vi "Normalizer.vi"(0 "Acc":u64[][](array[numeric]), 1 "m":dbl, 4 "p":dbl, 5 "Tamaño Sn":i32[](array[numeric]), 6 "Analysis 2":u16(ring) items=["Auto correlation A", "Auto correlation B", "Cross correlation AxB", "Cross correlation BxA"], 7 "AvgA":dbl, 10 "DataA":sgl[](array[numeric]), 11 "AvgB":dbl, 12 "DataB":sgl[](array[numeric])) -> (14 "g(k)":dbl[][](array[numeric]), 18 "s(k)":dbl[][](array[numeric]))   [LabVIEW 2015]
panel:
  out "X2Tau":dbl[][](array[numeric])
  out "X2i":dbl[][](array[numeric])
  out "element":i32
  out "size(s)":i32[](array[numeric])
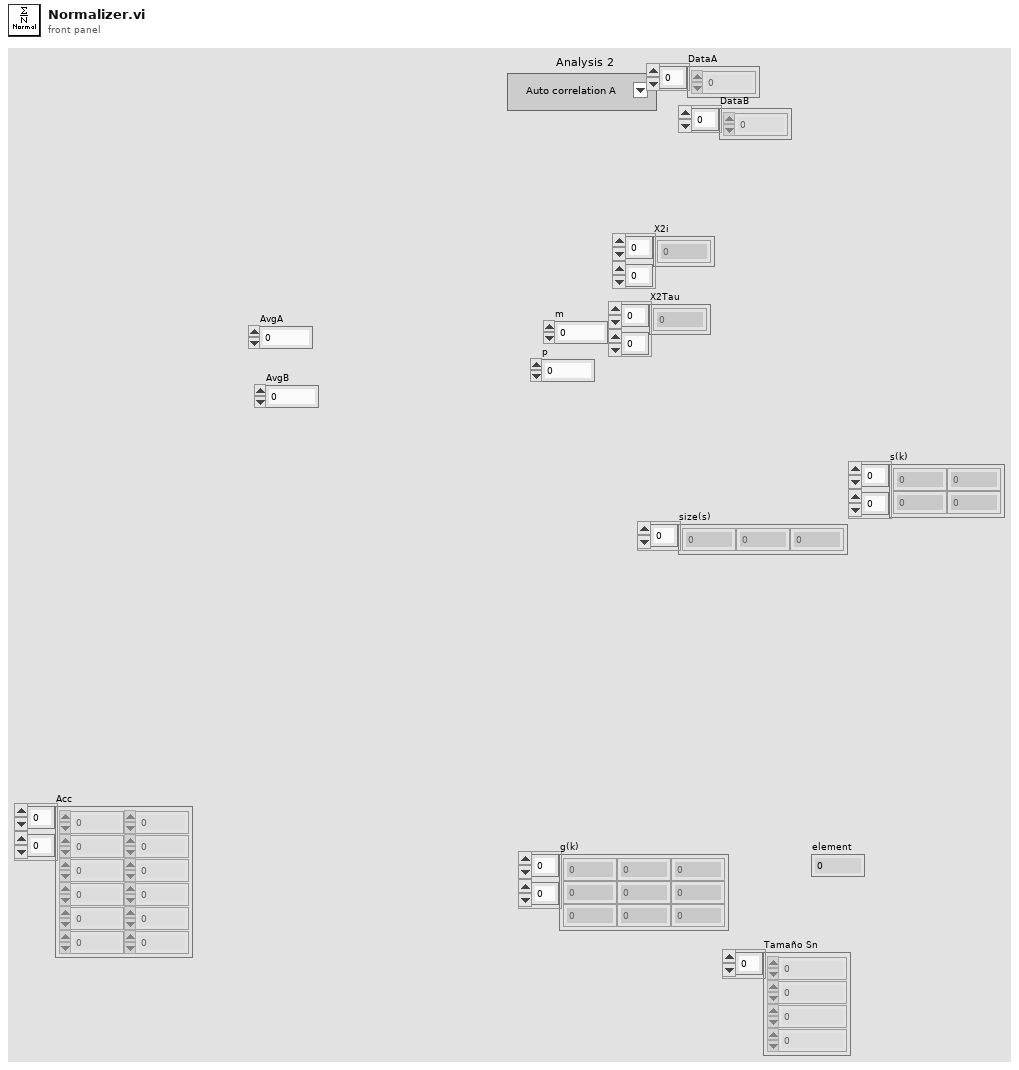
[diagram p1: front panel]
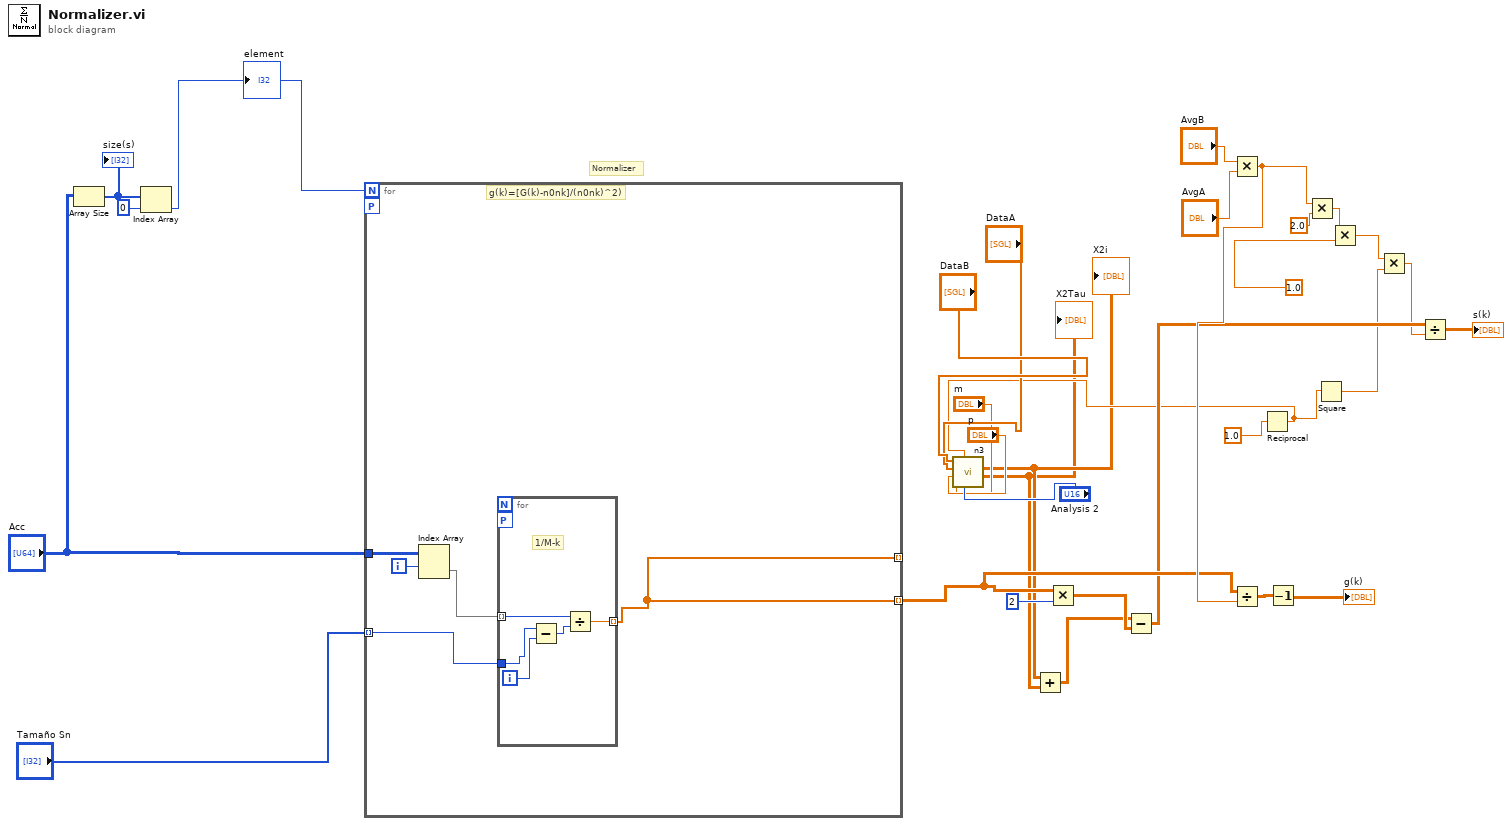
[diagram p0: block diagram]
diagram:
  # "Normalizer"
  n1 = Array Size(array="Acc") -> (size(s)=w28:i32[])
  "size(s)" <- w28
  n2 = Index Array(array=w28, index=0) -> (element=w30:i32)
  "element" <- w30
  n3 = for {
    N: w30 -> [_]
    tunnel: "Acc" -> [w34]
    tunnel: "Tamaño Sn" -> [w36] mode=indexing
    tunnel: [w32] -> w17 mode=indexing
    tunnel: [w32] -> _ mode=indexing
    workers-P: _ -> [_]
    i -> [w33]
    # "g(k)=[G(k)-n0nk]/(n0nk)^2)"
    n4 = Index Array(array=w34, index (row)=w33) -> (element=w35:u64[])  [unwired: 1 in]
    n5 = for {
      tunnel: [w41] -> w32 mode=indexing
      tunnel: w35 -> [w40] mode=indexing
      tunnel: w36 -> [w38]
      workers-P: _ -> [_]
      i -> [w37]
      # "1/M-k"
      n6 = Subtract(x=w38, y=w37) -> (x-y=w39:i32)
      n7 = Divide(x=w40, y=w39) -> (x/y=w41:dbl)
    }
  }
  n8 = Multiply(x=w17, y=2 ("index")) -> (x*y=w25:dbl[][])
  n9 = Multiply(x="AvgB", y="AvgA") -> (x*y=w21:dbl)
  n10 = Divide(x=w17, y=w21) -> (x/y=w23:dbl[][])
  n11 = Reciprocal(x=1.0) -> (1/x=w4:dbl)
  n12 = call "n3.vi"("Analysis"="Analysis 2", "beta"=w4, "m"="m", "P"="p", "Segmentation A"="DataA", "Segmentation B"="DataB") -> ("X2_tau"=w2:dbl[][], "X2_i"=w3:dbl[][])  [unwired: 4 in]
  "X2i" <- w3
  "X2Tau" <- w2
  n13 = Add(x=w3, y=w2) -> (x+y=w24:dbl[][])
  n14 = Subtract(x=w24, y=w25) -> (x-y=w14:dbl[][])
  n15 = Decrement(x=w23) -> (x-1=→"g(k)":dbl[][])
  n16 = Multiply(x=w21, y=2.0) -> (x*y=w16:dbl)
  n17 = Square(x=w4) -> (x^2=w6:dbl)
  n18 = Multiply(x=w16, y=1.0) -> (x*y=w7:dbl)
  n19 = Multiply(x=w7, y=w6) -> (x*y=w5:dbl)
  n20 = Divide(x=w14, y=w5) -> (x/y=→"s(k)":dbl[][])
